vi "Query.vi"(7 "Return":bool, 8 "error in (no error)":errorcluster, 10 "Command":string, 11 "PEU in":refnum<class "PEU.lvclass">) -> (0 "error out":errorcluster, 2 "read buffer":string, 3 "PEU out":refnum<class "PEU.lvclass">)   [LabVIEW 2020, in "PEU.lvlib" / "PEU.lvclass"]
uses:
  PEU.lvclass
  PEU.lvclass/PEU.ctl
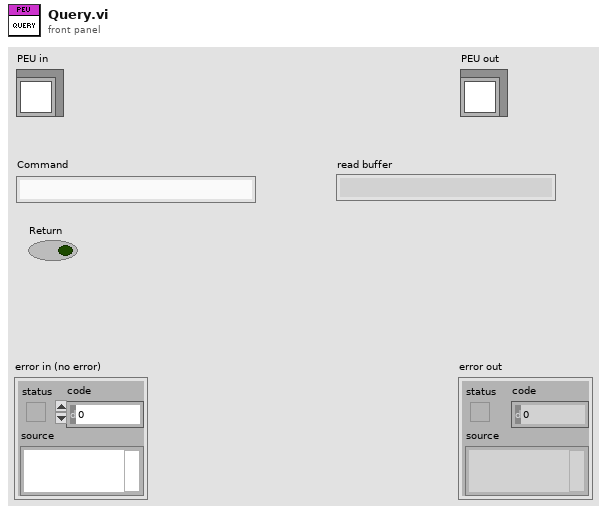
[diagram p1: front panel]
types:
  T1 = enum16{"Standard", "Buffered", "CRLF", "Immediate"}
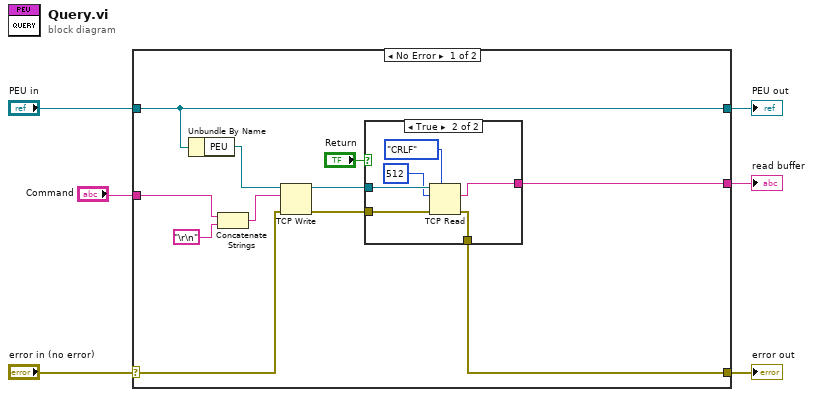
[diagram p0: block diagram]
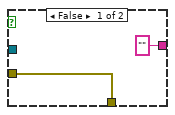
[diagram p2: hidden frame]
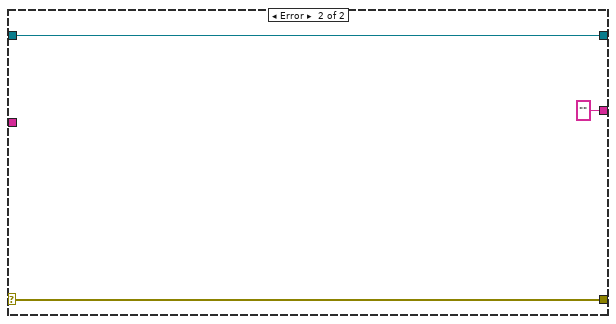
[diagram p3: hidden frame]
diagram:
  n1 = case shown="No Error" "error in (no error)" {
    selector: "error in (no error)" -> [w13 w28]
    tunnel: [w12 w28] -> w5
    tunnel: [w17 w27] -> w3
    tunnel: "PEU in" -> [w17 w27]
    tunnel: "Command" -> [w9 _]
    tunnel: [w10 "" ("data out")] -> w1
    frame No Error {
      n2 = Unbundle By Name(w17) -> ("PEU"=w16:refnum<k5>)
      n3 = Concatenate Strings(w9, "\r\n") -> (w7:string)
      n4 = TCP Write(connection ID=w16, data in=w7, error in (no error)=w13) -> (connection ID out=w15:refnum<k5>, error out=w14:errorcluster)  [unwired: 1 in, 1 out]
      n5 = case shown="True" "Return" {
        tunnel: w15 -> [_ w25]
        tunnel: w14 -> [w18 w24]
        tunnel: [w18 w23] -> w12
        tunnel: ["" ("data out") w21] -> w10
        frame False {
        }
        frame True {
          n6 = TCP Read(connection ID=w25, bytes to read=u32 512, error in (no error)=w24, 7:T1."CRLF" ("mode (standard)")) -> (data out=w21:string, error out=w23:errorcluster)  [unwired: 1 in, 1 out]
        }
      }
    }
    frame Error {
    }
  }
  "error out" <- w5
  "PEU out" <- w3
  "read buffer" <- w1
